vi "Main.vi"(11 "Module Admin":refnum<class "Delacor_lib_QMH_Module Admin.lvclass">) -> ()   [LabVIEW 2020, in "UI.lvlib"]
doc: "This template is based off of the Queued Message Handler design pattern and the Queued Message Handler project template that ships with LabVIEW.\n\nThe main difference is that the queue is private to this module and communication between modules is performed via Broadcast and Request events.\n\nRequest events are wrapped in public API methods and are handled in the Event Handling Loop (EHL) of this VI. Any module can register for Broadcast events sent by this module. The EHL generates messages based on user interface actions.\n\nThe Message Handling Loop (MHL) processes messages generated by the EHL, or by other messages. The messages are string values, so new messages can be added easily to the Message Cases case structure in the MHL. Each message cluster can also provide an optional value for Message Data, which is a variant that can be converted to whatever message-specific data is required.\n_____\nBased on DQMH Dev Tools: Project Template 7.1.1.1528."
uses:
  UI.lvlib
  <vilib>/Delacor/Delacor QMH/Libraries/Module Admin_class/Delacor_lib_QMH_Module Admin.lvclass
  <vilib>/Delacor/Delacor QMH/Libraries/Message Queue_class/Delacor_lib_QMH_Message Queue.lvclass/Delacor_lib_QMH_Message Queue.ctl
  <vilib>/Delacor/Delacor QMH/Libraries/Module Admin_class/Delacor_lib_QMH_Module Admin.lvclass/Delacor_lib_QMH_Module Admin.ctl
  <vilib>/Delacor/Delacor QMH/Libraries/Message Queue_class/Delacor_lib_QMH_Message Queue.lvclass
  Module Data--cluster.ctl
  <vilib>/Delacor/Delacor QMH/Libraries/Message Queue_class/Delacor_lib_QMH_Enqueue Message (Single).vi
  Stop Argument--cluster.ctl
  NI_DAQ/Libraries/NI DAQ/NI DAQ.lvlib
  NI_DAQ/Libraries/NI DAQ/Controls/AI config parameters--cluster.ctl
  <vilib>/Utility/sysdir.llb/System Directory Type.ctl
  <vilib>/Delacor/Delacor QMH/Libraries/Message Queue_class/Delacor_lib_QMH_Enqueue Message (Array).vi
panel:
  out "Remaining time":string caption="Tiempo restante"
  in  "Sample time":i32=1 caption="Muestreo (seg)"
  in  "Acq Time":dbl=1.0 caption="Tiempo (hrs)"
  in  "Log":bool
  in  "Stop Button":bool
  in  "Acquire":bool
  out "Temperatura":dbl format="%#_g °C"
  out "Voltage graph":dbl(graph)
  out "Status":string caption="Estado del sistema"
  out "Adquiriendo":bool
  out "DAQ":bool
  in  "Simulate MHL Error":bool
  in  "Simulate EHL Error":bool
  in  "Settings Button":bool
  in  "Exit Button":bool
  in  "Help Button":bool
  out "error out":errorcluster
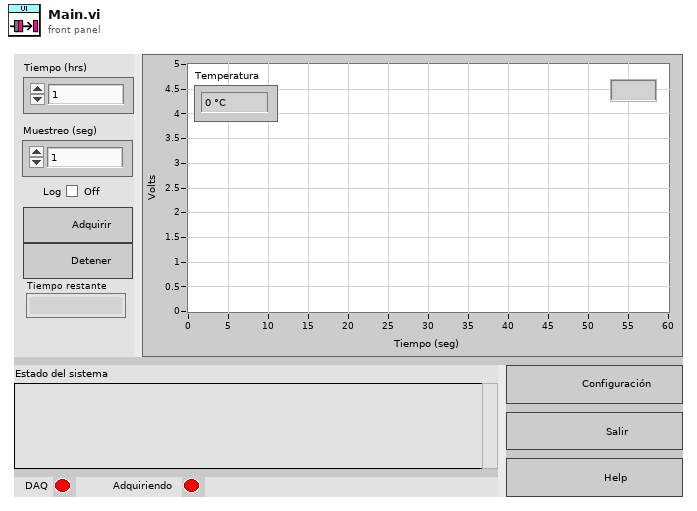
[diagram p1: front panel]
types:
  T1 = typedef "NI DAQ.lvlib/Broadcast Events--cluster.ctl" = cluster{"Module Did Init":refnum<user-event>, "Status Updated":refnum<user-event>, "Error Reported":refnum<user-event>, "Module Did Stop":refnum<user-event>, "Update Module Execution Status":refnum<user-event>, "Digital data acquired":refnum<user-event>, "Device connected":refnum<user-event>, "Connection failed":refnum<user-event>, "Analog data acquired":refnum<user-event>, "Counter data acquired":refnum<user-event>, "Temperature data acquired":refnum<user-event>}
  T2 = typedef "UI.lvlib/Request Events--cluster.ctl" = cluster{"Stop Module":refnum<user-event>, "Show Panel":refnum<user-event>, "Hide Panel":refnum<user-event>, "Get Module Execution Status":refnum<user-event>, "Show Diagram":refnum<user-event>}
  T3 = typedef "UI.lvlib/Module Data--cluster.ctl" = cluster{"Status":string, "DAQ module ID":i32, "DAQ Device":tag, "Start time":timestamp, "Stop time":timestamp, "Log file ref":refnum<file>}
  T4 = enum32{"invalid lock state", "Not Locked", "Locked (No Password)", "Password-protected"}
  T5 = typedef "UI.lvlib/Stop Argument--cluster.ctl" = cluster{"Origin":string, "Exit via Stop Module Req?":bool, "Wait for Module to stop?":bool}
  T6 = enum32{"Invalid", "Standard", "Closed", "Hidden", "Minimized", "Maximized"}
  T7 = cluster{"max value":dbl, "min value":dbl, "type":i32, "CJC source":i32, "cjc channel":refnum<k21>, "CJC value":dbl}
  T8 = typedef "NI DAQ.lvlib/AI config parameters--cluster.ctl" = cluster{"Terminal configuration":i32, "min value":dbl, "max value":dbl}
  T9 = enum16{"open", "replace", "create", "open or create", "replace or create", "replace or create with confirmation"}
  T10 = typedef "System Directory Type.ctl" = i32
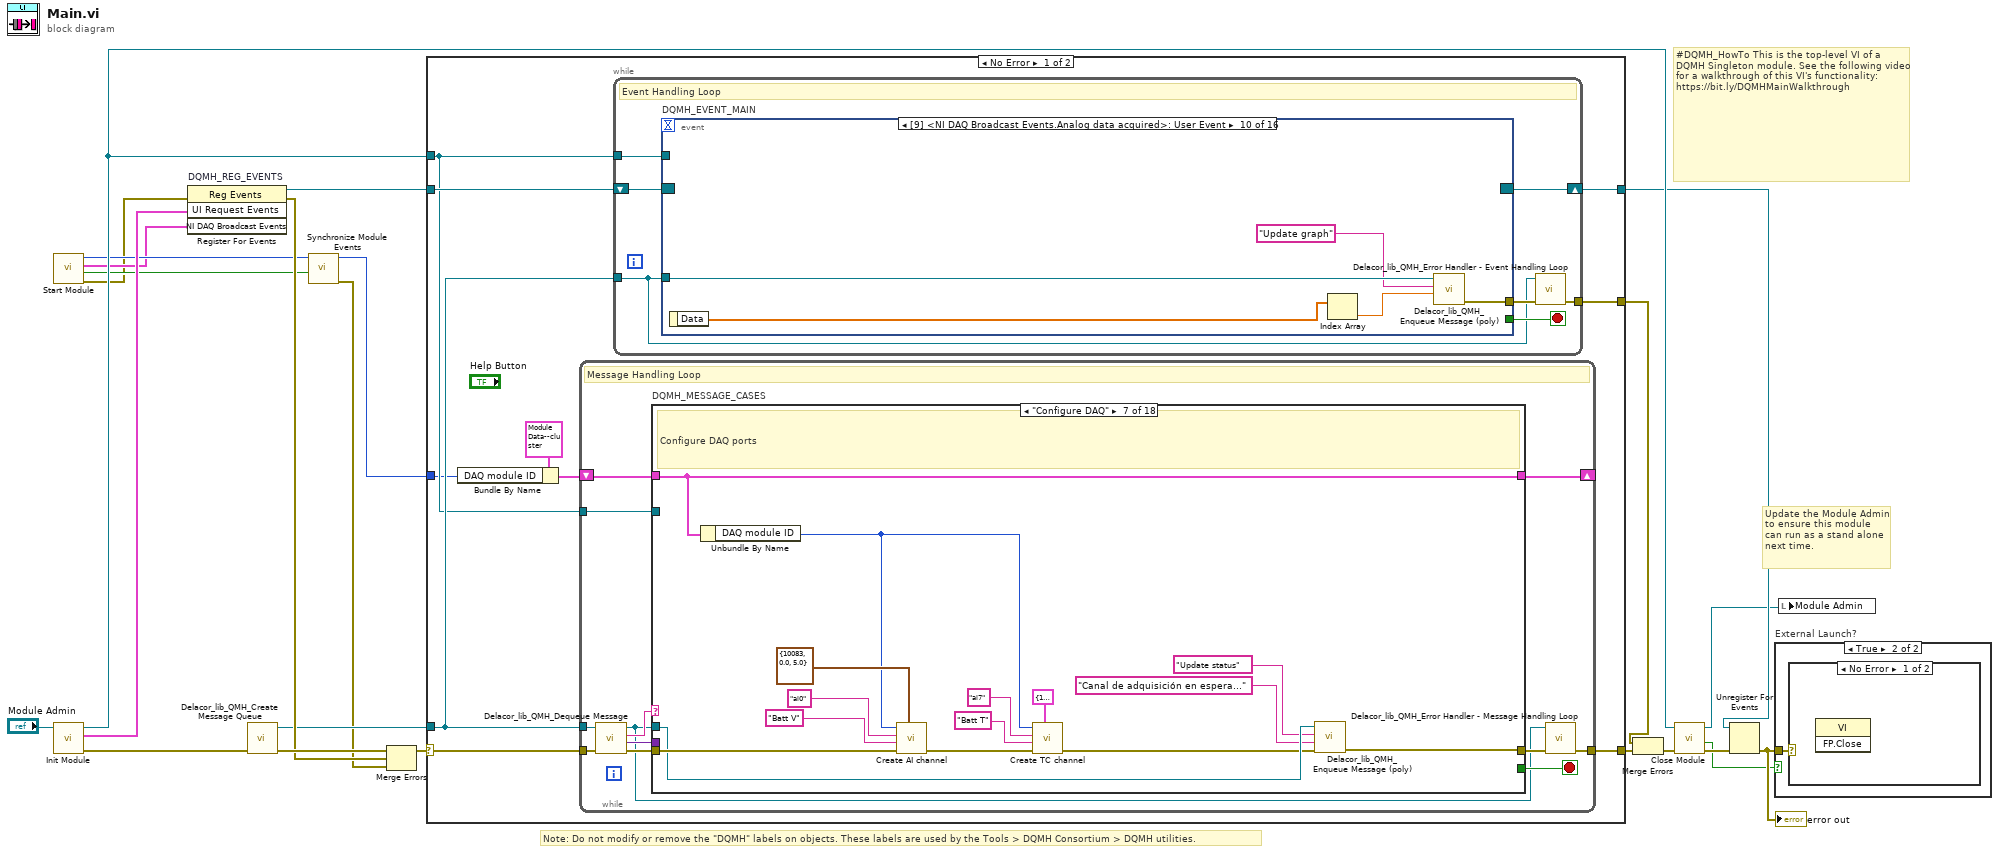
[diagram p0: block diagram]
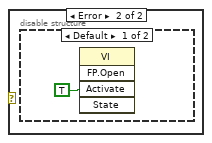
[diagram p3: hidden frame]
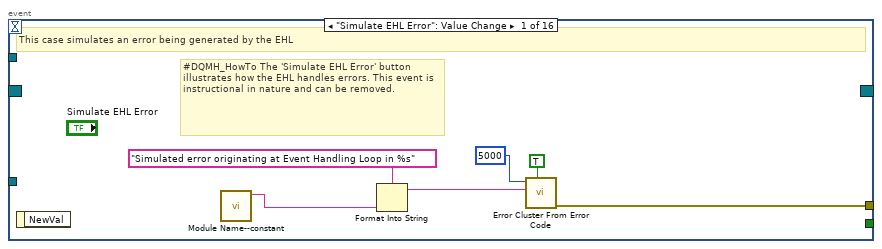
[diagram p5: hidden frame]
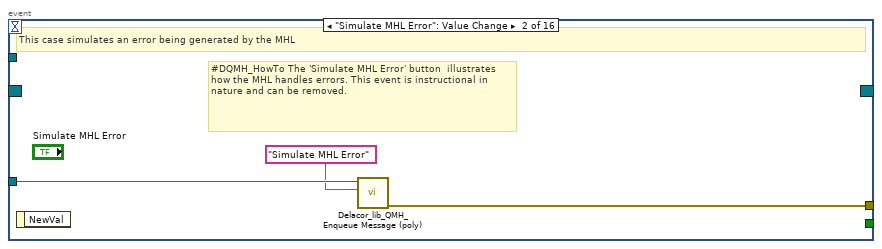
[diagram p6: hidden frame]
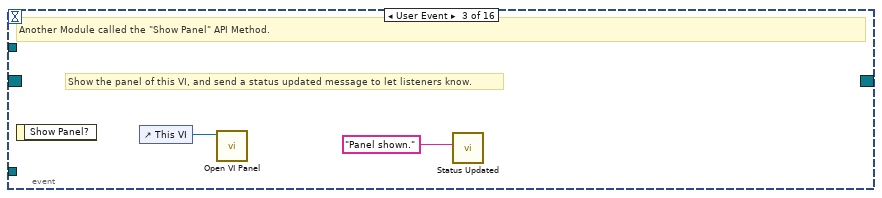
[diagram p7: hidden frame]
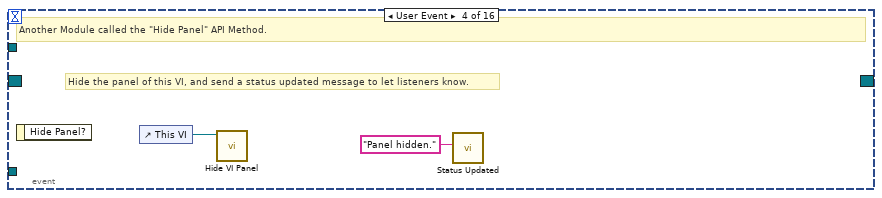
[diagram p8: hidden frame]
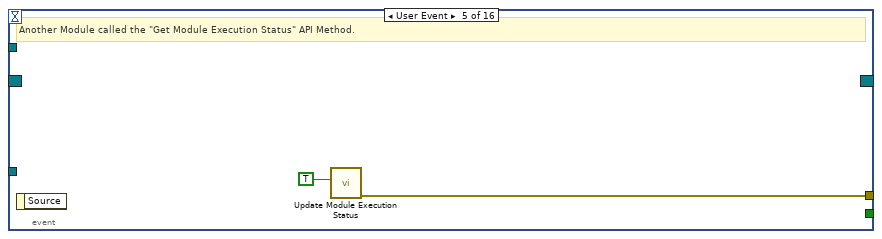
[diagram p9: hidden frame]
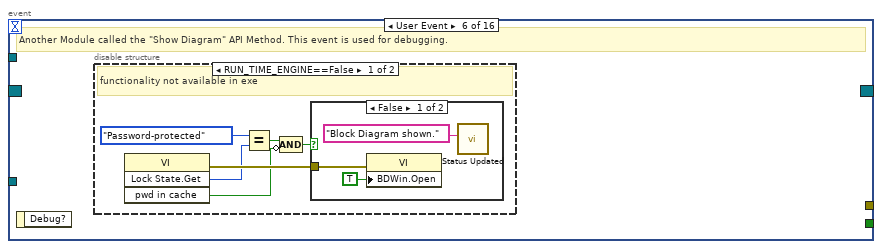
[diagram p10: hidden frame]
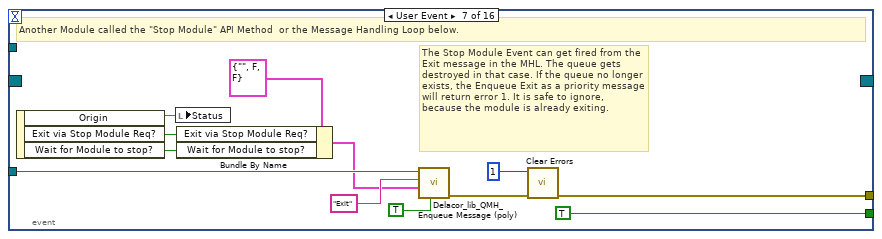
[diagram p13: hidden frame]
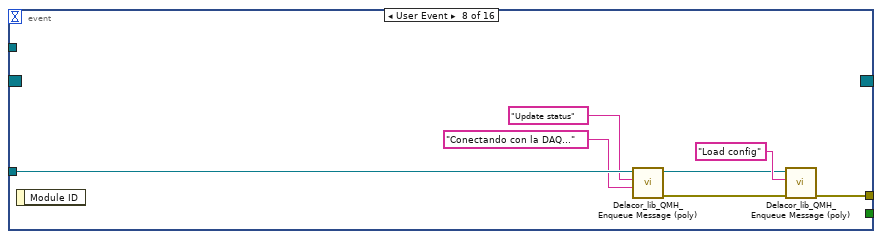
[diagram p14: hidden frame]
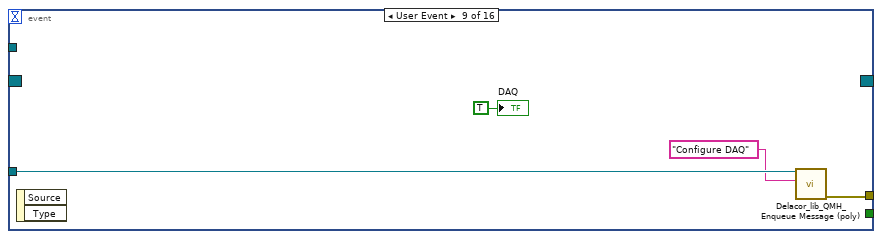
[diagram p15: hidden frame]
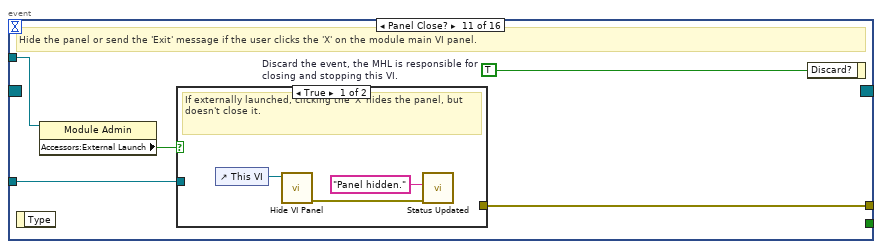
[diagram p16: hidden frame]
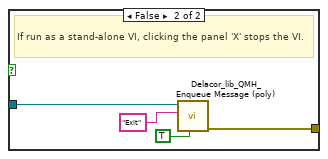
[diagram p17: hidden frame]
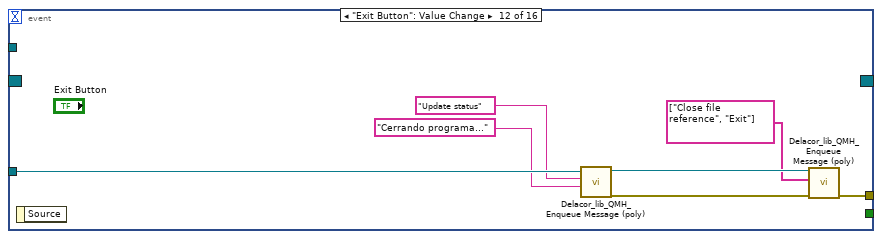
[diagram p18: hidden frame]
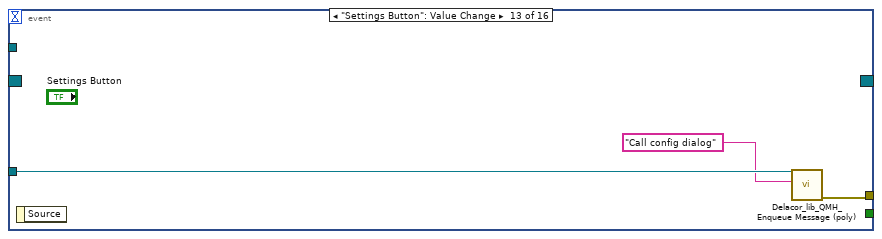
[diagram p19: hidden frame]
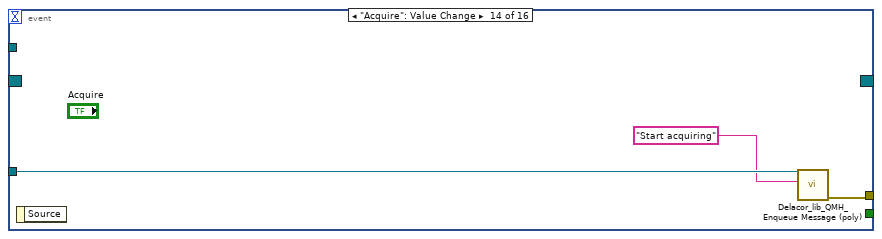
[diagram p20: hidden frame]
diagram:
  # "#DQMH_HowTo This is the top-level VI of a DQMH Singleton module. See the following video for a walkthrough of this VI's functionality: https://bit.ly/DQMHMainWalkthrough"
  # "Note: Do not modify or remove the \"DQMH\" labels on objects. These labels are used by the Tools > DQMH Consortium > DQMH utilities."
  # "Update the Module Admin to ensure this module can run as a stand alone next time."
  n1 = call "Start Module.vi"() -> ("error out"=w2:errorcluster, "Wait for Event Sync?"=w5:bool, "NI DAQ Broadcast Events"=w4:T1, "Module ID"=w6:i32)  [unwired: 8 in]
  n2 = call "Init Module.vi"("Singleton Module Admin in"="Module Admin") -> ("error out"=w22:errorcluster, "UI Request Events"=w11:T2, "Singleton Module Admin out"=w14:refnum<class "Delacor_lib_QMH_Module Admin.lvclass">)  [unwired: 8 in]
  n3 = register-events "DQMH_REG_EVENTS"(error in=w2, w11, w4) -> (reference out=w12:refnum<event-registration>, error out=w15:errorcluster)  [unwired: 1 in]
  n4 = call <vilib>:"Delacor_lib_QMH_Create Message Queue.vi"("error in"=w22) -> ("error out"=w17:errorcluster, "Message Queue"=w10:refnum<class "Delacor_lib_QMH_Message Queue.lvclass">)  [unwired: 9 in]
  n5 = call "Synchronize Module Events.vi"("Wait for Event Sync?"=w5, "Module ID in"=w6) -> ("error out"=w3:errorcluster, "Module ID out"=w1:i32)  [unwired: 8 in]
  n6 = Merge Errors(w17, w15, w3) -> (w16:errorcluster)
  n7 = case shown="No Error" w16 {
    selector: w16 -> [w31 w466]
    tunnel: [w33 w465] -> w23
    tunnel: [w30 w464] -> w13
    tunnel: w12 -> [w29 w464]
    tunnel: w10 -> [w28 w459]
    tunnel: [w32 _] -> w20
    tunnel: w14 -> [w27 w460]
    tunnel: w1 -> [w24 w458]
    frame No Error {
      n8 = Bundle By Name(cluster=T3 {"Status"="", "DAQ module ID"=0, "DAQ Device"="", "Start time"=timestamp(0 s since 1904-01-01), "Stop time"=timestamp(0 s since 1904-01-01), "Log file ref"=refnum} ("Data Cluster"), "DAQ module ID"=w24) -> (w26:T3)
      n9 = while {
        tunnel: w28 -> [w127]
        shift-right: [w135] -> _
        shift-left: w26 -> [w136]
        tunnel: w31 -> [w138]
        tunnel: [w130] -> w33
        tunnel: w27 -> [w131]
        stop <- w134 stop-if-true
        # "Message Handling Loop"
        n10 = call-dynamic "Delacor_lib_QMH_Dequeue Message.vi"("error in"=w138, "Message Queue in"=w127) -> ("error out"=w137:errorcluster, "Message Data"=w132:variant, "Message"=w133:string, "Message Queue out"=w128:refnum<class "Delacor_lib_QMH_Message Queue.lvclass">)  [unwired: 6 in]
        n11 = case "DQMH_MESSAGE_CASES" shown="\"Configure DAQ\"" w133 {
          selector: w133 -> [_ _ _ _ _ _ _ _ _ _ _ _ _ _ _ _ _ w453]
          tunnel: w128 -> [_ _ _ w176 w203 w221 w244 w264 w279 w296 w351 w380 _ _ _ w417 w441 _]
          tunnel: w137 -> [w162 w166 w169 w182 w204 w218 w250 w255 w274 w302 w355 w384 w396 w398 w413 w424 w447 w456]
          tunnel: [w161 w166 w168 w180 w198 w224 w245 w265 w280 w299 w352 w381 w389 w397 w412 w420 w442 w457] -> w129
          tunnel: w136 -> [w152 w165 w167 w181 w205 w220 w249 w267 w281 w286 w343 w383 w388 w399 w410 w419 w433 w454]
          tunnel: [w152 w165 w167 w170 w205 w219 w249 w266 w281 w286 w342 w383 w387 w399 w410 w419 w433 w454] -> w135
          tunnel: [_ _ _ _ _ _ _ _ _ _ _ _ _ _ _ _ w440 _] -> w134
          tunnel: w132 -> [_ _ _ _ _ _ _ _ _ w301 _ _ w394 _ _ w418 w439 _]
          tunnel: w131 -> [w153 _ _ _ _ _ _ _ _ _ _ _ _ _ _ w416 w434 _]
          frame "Initialize" {
            w140 = FALSE ("DAQ")
            # "Initialize - Any operation that needs to be done before the module can receive messages. Synchronize Caller Events.vi will inform Start Module.vi that the module has launched and is ready to receive messages. Module Did Init.vi will broadcast that the module initialized."
            n12 = call "Synchronize Caller Events.vi"("error in"=w162, "Singleton Module Admin in"=w153) -> ("error out"=w145:errorcluster, "Singleton Module Admin out"=w149:refnum<class "Delacor_lib_QMH_Module Admin.lvclass">)  [unwired: 8 in]
            n13 = property on="Property Node" class="Module Admin"(reference=w149) -> ("Accessors:External Launch"=w157:bool)  [unwired: 1 in, 2 out]
            n14 = property on="Voltage graph" class="WFChart (strict)"(error in=w145, "History Data"=dbl[] [], "XScale.RngStart"=0.0 ("X Scale.Range:Start"), "XScale.Maximum"=60.0 ("X Scale.Range:Maximum"), "XScale.Increment"=1.0 ("X Scale.Range:Increment")) -> (error out=w139:errorcluster)  [unwired: 1 in, 1 out]
            n15 = Select(t=T6."Hidden" ("State"), s=w157, f=T6."Standard" ("State")) -> (s? t:f=w154:T6)
            n16 = call "Module Name--constant.vi"() -> ("Module Name"=w160:string)  [unwired: 11 in]
            n17 = property on="Property Node" class="VI"("Front Panel.Title"=w160) -> (reference out=w159:refnum<vi>, error out=w164:errorcluster)  [unwired: 2 in]
            n18 = invoke on="Invoke Node" class="VI" method="FP.Open"(reference=w159, error in=w164, "State"=w154) -> (reference out=w158:refnum<vi>, error out=w163:errorcluster)  [unwired: 2 in, 3 out]
            n19 = property on="Adquiriendo" class="Bool (strict)"(error in=w139, "Value"=w140) -> ()  [unwired: 1 in, 2 out]
            n20 = property on="DAQ" class="Bool (strict)"(error in=w139, "Value"=w140) -> (error out=w148:errorcluster)  [unwired: 1 in, 1 out]
            n21 = control-ref of="This VI"() -> (w146:refnum<vi>)
            n22 = invoke on="Invoke Node" class="VI" method="FP.Center"(reference=w158, error in=w163) -> ()  [unwired: 1 in, 3 out]
            n23 = invoke class="VI" method="Default Vals.Reinit All"(reference=w146, error in=w148) -> (error out=w147:errorcluster)  [unwired: 1 in, 2 out]
            n24 = call "Module Name--constant.vi"() -> ("Module Name"=w150:string)  [unwired: 11 in]
            n25 = call "Module Did Init.vi"("error in"=w147, "Initialized?"=TRUE, "Origin"=w150) -> ("error out"=w161:errorcluster)  [unwired: 8 in]
          }
          frame "---Module Specific---" {
            # "Separator -- The following cases handle messages specific to this Module."
          }
          frame "---Copy This Frame---" {
            # "Duplicate this frame when creating new messages.  Change this comment in the duplicated frame to describe this message."
            n26 = Merge Errors(w169) -> (w168:errorcluster)
          }
          frame "Load config" {
            # "Try to load data from config.ini. If file is non existent, call configuration dialog, otherwise configure DAQ and enter idle status."
            n27 = call "Load config.vi"("error in (no error)"=w182, "Data Cluster in"=w181) -> ("error out"=w172:errorcluster, "Call config dialog?"=w179:bool, "Data Cluster out"=w170:T3)  [unwired: 7 in]
            n28 = case shown="True" w179 {
              tunnel: ["Validate DAQ" "Call config dialog"] -> w178
              tunnel: ["Configuración cargada. Validando..." "DAQ no conectada. Lanzando diálogo de configuración."] -> w173
              tunnel: w172 -> [w187 w192]
              tunnel: [w186 w191] -> w171
              tunnel: w170 -> [w185 _]
              frame False {
                # "Connection successful. Validate DAQ."
                n29 = Unbundle By Name(w185) -> ("DAQ module ID"=w184:i32, "DAQ Device"=w183:tag)
                n30 = call "Set device name.vi"("error in"=w187, "Device name"=w183, "Module ID"=w184) -> ("error out"=w186:errorcluster)  [unwired: 8 in]
              }
              frame True {
                w190 = -200220  # Invalid DAQ name reference
                # "Connection failed. Send config dialog"
                n31 = call <vilib>:"Clear Errors.vi"("error in (no error)"=w192, "specific error code to clear (0: all)"=w190) -> ("error out"=w191:errorcluster)  [unwired: 4 in, 1 out]
              }
            }
            n32 = call-poly <vilib>:"Delacor_lib_QMH_Enqueue Message (poly).vi"("error in"=w171, "Message Data"=w173, "Message"="Update status", "Message Queue in"=w176) -> ("error out"=w177:errorcluster, "Message Queue out"=w175:refnum<class "Delacor_lib_QMH_Message Queue.lvclass">)  [unwired: 6 in]
            n33 = call-poly <vilib>:"Delacor_lib_QMH_Enqueue Message (poly).vi"("error in"=w177, "Message"=w178, "Message Queue in"=w175) -> ("error out"=w180:errorcluster)  [unwired: 7 in, 1 out]
          }
          frame "Validate DAQ" {
            # "Identify DAQ Model and validate connection."
            n34 = Unbundle By Name(w205) -> ("DAQ module ID"=w195:i32)
            n35 = call "Get device model.vi"("error in"=w204, "Module ID"=w195) -> ("error out"=w197:errorcluster, "Device model"=w200:string)  [unwired: 7 in, 1 out]
            n36 = Empty String/Path?(string/path=w200) -> (empty?=w199:bool)
            n37 = case shown="False" w199 {
              tunnel: [w210 "La tarjeta DAQ conectada no es válida."] -> w201
              tunnel: w200 -> [w209 _]
              tunnel: w197 -> [w208 w213]
              tunnel: [w207 w213] -> w196
              tunnel: w195 -> [w206 _]
              frame False {
                # "DAQ Model not empty. Validate connection."
                n38 = Format Into String(format string="DAQ %s encontrada.", w209) -> (resulting string=w210:string)  [unwired: 2 in, 1 out]
                n39 = call "Validate connection.vi"("error in"=w208, "Module ID"=w206) -> ("error out"=w207:errorcluster)  [unwired: 7 in, 2 out]
              }
              frame True {
                # "DAQ Model string empty."
              }
            }
            n40 = call-poly <vilib>:"Delacor_lib_QMH_Enqueue Message (poly).vi"("error in"=w196, "Message Data"=w201, "Message"="Update status", "Message Queue in"=w203) -> ("error out"=w198:errorcluster)  [unwired: 6 in, 1 out]
          }
          frame "Call config dialog" {
            n41 = property on="DAQ" class="Bool (strict)"(error in=w218, "Value"=FALSE ("DAQ")) -> (error out=w216:errorcluster)  [unwired: 1 in, 1 out]
            n42 = Unbundle By Name(w220) -> ("DAQ module ID"=w214:i32)
            n43 = call "Stop continuous acquisition.vi"("error in"=w216, "Module ID"=w214) -> ("error out"=w215:errorcluster)  [unwired: 9 in]
            n44 = call "Config dialog.vi"("error in (no error)"=w215, "DAQ module ID"=w214) -> ("error out"=w225:errorcluster, "Cancelled?"=w223:bool, "DAQmx Device Name out"=w222:tag)  [unwired: 7 in]
            n45 = case shown="False" w223 {
              tunnel: w225 -> [w227 w235]
              tunnel: [w233 w235] -> w224
              tunnel: w222 -> [w228 _]
              tunnel: w221 -> [w232 _]
              tunnel: w220 -> [w230 w234]
              tunnel: [w229 w234] -> w219
              frame False {
                # "Save config and try to connect."
                n46 = call "Save config.vi"("error in (no error)"=w227, "DAQ Device Name"=w228) -> ("error out"=w226:errorcluster)  [unwired: 9 in]
                n47 = Bundle By Name(cluster=w230, "DAQ Device"=w228) -> (w229:T3)
                n48 = call-poly <vilib>:"Delacor_lib_QMH_Enqueue Message (poly).vi"("error in"=w226, "Message"="Load config", "Message Queue in"=w232) -> ("error out"=w233:errorcluster)  [unwired: 7 in, 1 out]
              }
              frame True {
                # "Dialog was cancelled. Do nothing."
              }
            }
          }
          frame "Configure DAQ" {
            # "Configure DAQ ports"
            n49 = Unbundle By Name(w249) -> ("DAQ module ID"=w239:i32)
            n50 = call "Create AI channel.vi"("Config params"=T8 {"Terminal configuration"=10083, "min value"=0.0, "max value"=5.0}, "error in"=w250, "Channel name"="Batt V", "Physical channel"="ai0", "Module ID"=w239) -> ("error out"=w241:errorcluster)  [unwired: 6 in]
            n51 = call "Create TC channel.vi"("TC Config"=T7 {"max value"=100.0, "min value"=0.0, "type"=10073, "CJC source"=10116, "cjc channel"="", "CJC value"=23.0}, "error in"=w241, "Channel name"="Batt T", "Physical channel"="ai7", "Module ID"=w239) -> ("error out"=w240:errorcluster)  [unwired: 6 in]
            n52 = call-poly <vilib>:"Delacor_lib_QMH_Enqueue Message (poly).vi"("error in"=w240, "Message Data"="Canal de adquisición en espera..." ("Message"), "Message"="Update status", "Message Queue in"=w244) -> ("error out"=w245:errorcluster)  [unwired: 6 in, 1 out]
          }
          frame "Start acquiring" {
            w270 = 1000  # To ms
            # "Begin continuous acquisition of analog input channel."
            n53 = Unbundle By Name(w267) -> ("DAQ module ID"=w252:i32)
            n54 = Multiply(x="Sample time", y=w270) -> (x*y=w251:i32)
            n55 = call "Start continuous AI.vi"("error in"=w255, "Acq type"=enum16{"Single", "Multiple"}."Single" ("Samples"), "Timeout"=w251, "Module ID"=w252) -> ("error out"=w253:errorcluster)  [unwired: 7 in]
            n56 = local read "Acq Time"() -> (w260:dbl)
            n57 = Get Date/Time In Seconds() -> (seconds since 1Jan1904=w258:timestamp)
            n58 = property on="Voltage graph" class="WFChart (strict)"(error in=w253, "History Data"=dbl[] []) -> (error out=w269:errorcluster)  [unwired: 1 in, 1 out]
            n59 = Multiply(x=w260, y=3600.0) -> (x*y=w257:dbl)
            n60 = Add(x=w258, y=w257) -> (x+y=w256:timestamp)
            n61 = Bundle By Name(cluster=w267, "Start time"=w258, "Stop time"=w256) -> (w266:T3)
            n62 = call-poly <vilib>:"Delacor_lib_QMH_Enqueue Message (poly).vi"("error in"=w269, "Message Data"="Adquisición en progreso..." ("Message"), "Message"="Update status", "Message Queue in"=w264) -> ("error out"=w265:errorcluster)  [unwired: 6 in, 1 out]
            "Adquiriendo" <- TRUE ("Adquiriendo")
          }
          frame "Stop acquisition" {
            n63 = Unbundle By Name(w281) -> ("DAQ module ID"=w272:i32)
            n64 = call "Stop continuous AI.vi"("error in"=w274, "Module ID"=w272) -> ("error out"=w273:errorcluster)  [unwired: 9 in]
            n65 = property on="Adquiriendo" class="Bool (strict)"(error in=w273, "Value"=FALSE ("Adquiriendo")) -> (error out=w276:errorcluster)  [unwired: 1 in, 1 out]
            n66 = call-poly <vilib>:"Delacor_lib_QMH_Enqueue Message (poly).vi"("error in"=w276, "Message Data"="Adquisitión detenida" ("Message"), "Message"="Update status", "Message Queue in"=w279) -> ("error out"=w280:errorcluster)  [unwired: 6 in, 1 out]
          }
          frame "Update graph" {
            w293 = 3600.0  # h to sec
            # "Updates graph contents and checks wether Log to file is active. If Log is set to True, write a new row to Log file."
            n67 = Variant To Data(error in=w302, type=0.0, Variant=w301) -> (data=w294:dbl, error out=w288:errorcluster)
            "Voltage graph" <- w294
            n68 = Unbundle By Name(w286) -> ("Stop time"=w289:timestamp, "Start time"=w290:timestamp)
            n69 = Unbundle By Name(w286) -> ("DAQ module ID"=w285:i32)
            n70 = Get Date/Time In Seconds() -> (seconds since 1Jan1904=w295:timestamp)
            n71 = Subtract(x=w295, y=w290) -> (x-y=w298:dbl)
            n72 = call "Read TC.vi"("error in"=w288, "N samples"=10, "Reading Type"=enum16{"Single", "Average"}."Average", "Module ID"=w285) -> ("error out"=w287:errorcluster, "Temperature"=w282:dbl)  [unwired: 5 in, 1 out]
            "Temperatura" <- w282
            n73 = Multiply(x="Acq Time", y=w293) -> (x*y=w291:dbl)
            n74 = Less Or Equal?(x=w298, y=w291) -> (x <= y?=w297:bool)
            n75 = case shown="True" w297 {
              tunnel: w287 -> [w304 w327]
              tunnel: [w308 w325] -> w299
              tunnel: w286 -> [w318 w324]
              tunnel: w296 -> [w314 _]
              tunnel: w295 -> [w311 w322]
              tunnel: w294 -> [_ w323]
              tunnel: w289 -> [_ w321]
              tunnel: w282 -> [_ w319]
              frame False {
                # "Total acquisition time reached. Stop acquisition"
                n76 = Unbundle By Name(w318) -> ("DAQ module ID"=w317:i32)
                n77 = property on="Adquiriendo" class="Bool (strict)"(error in=w304, "Value"=FALSE ("Adquiriendo")) -> (error out=w303:errorcluster)  [unwired: 1 in, 1 out]
                n78 = Format Date/Time String(seconds (now)=w311) -> (date/time string=w310:string)  [unwired: 2 in]
                n79 = call "Stop continuous acquisition.vi"("error in"=w303, "Module ID"=w317) -> ("error out"=w316:errorcluster)  [unwired: 9 in]
                n80 = Format Into String(format string="Adquisición completada en %s.", w310) -> (resulting string=w309:string)  [unwired: 2 in, 1 out]
                n81 = One Button Dialog(message=w309) -> ()  [unwired: 1 in, 1 out]
                n82 = call-poly <vilib>:"Delacor_lib_QMH_Enqueue Message (poly).vi"("error in"=w316, "Message Data"=w309, "Message"="Update status", "Message Queue in"=w314) -> ("error out"=w315:errorcluster, "Message Queue out"=w307:refnum<class "Delacor_lib_QMH_Message Queue.lvclass">)  [unwired: 6 in]
                n83 = call-poly <vilib>:"Delacor_lib_QMH_Enqueue Message (poly).vi"("error in"=w315, "Message"="Close file reference", "Message Queue in"=w307) -> ("error out"=w308:errorcluster)  [unwired: 7 in, 1 out]
              }
              frame True {
                # "Total acquisition time not reached yet. Keep acquiring."
                n84 = call "Get remaining time.vi"("Stop time"=w321, "Curent time"=w322) -> ("Remaining time"=→"Remaining time":string)  [unwired: 9 in]
                n85 = case shown="True" "Log" {
                  tunnel: w327 -> [w328 w341]
                  tunnel: [w328 w336] -> w325
                  tunnel: w324 -> [_ w340]
                  tunnel: w323 -> [_ w331]
                  tunnel: w322 -> [_ w339]
                  tunnel: w319 -> [_ w329]
                  frame False {
                    # "Not logging. Do nothing."
                  }
                  frame True {
                    # "Log to file"
                    n86 = Unbundle By Name(w340) -> ("Log file ref"=w334:refnum<file>)
                    n87 = Get Date/Time String(date format (0)=enum16{"short", "long", "abbreviated"}."short", seconds (now)=w339, want seconds? (F)=TRUE) -> (date string=w333:string, time string=w332:string)
                    n88 = Format Into String(format string="%s %s,%0.6f,%0.2f\n", w333, w332, w331, w329) -> (resulting string=w335:string)  [unwired: 2 in, 1 out]
                    n89 = Write to Text File(file (use dialog)=w334, text=w335, error in=w341) -> (error out=w336:errorcluster)  [unwired: 1 in, 2 out]
                  }
                }
              }
            }
          }
          frame "Open file reference" {
            w347 = T10 2 items=["User Home"=0, "User Desktop"=1, "User Documents"=2, "User Application Data"=3, "User Preferences"=4, "User Temporary"=5, "Public Documents"=6, "Public Application Data"=7, "Public Preferences"=8, "Public Cache"=13, "System Core Libraries"=9, "System Installed Libraries"=10, "Application Files"=11, "Boot Volume Root"=12] ("system directory type")
            n90 = call <vilib>:"Get System Directory.vi"("system directory type"=w347) -> ("system directory"=w346:path)  [unwired: 10 in]
            n91 = call "File Dialog"("start path"=w346, "error in"=w355, "pattern (all files)"="*.csv") -> ("selected path"=w345:path, "cancelled"=w354:bool, "error out"=w344:errorcluster)  [unwired: 9 in, 1 out]
            n92 = case shown="False" w354 {
              tunnel: [w359 w374] -> w353
              tunnel: ["Registro de datos iniciado." ("Message") "Registro de datos cancelado." ("Message")] -> w349
              tunnel: w345 -> [w366 _]
              tunnel: w344 -> [w367 w369]
              tunnel: w343 -> [w361 w371]
              tunnel: [w360 w371] -> w342
              frame False {
                # "Dialog not cancelled. Open file reference."
                n93 = Open/Create/Replace File(file path (use dialog)=w366, error in=w367, operation (0:open)=T9."replace or create", access (0:read/write)=enum16{"read/write", "read-only", "write-only"}."write-only") -> (refnum out=w358:refnum<file>, error out=w365:errorcluster)  [unwired: 2 in, 1 out]
                n94 = Write to Text File(file (use dialog)=w358, text="Timestamp,Voltaje, Temperatura\n", error in=w365) -> (refnum out=w356:refnum<file>, error out=w359:errorcluster)  [unwired: 1 in, 1 out]
                n95 = Bundle By Name(cluster=w361, "Log file ref"=w356) -> (w360:T3)
              }
              frame True {
                w370 = 43  # Dialog cancelled
                # "Dialog was cancelled. Set Log flag to False."
                n96 = call <vilib>:"Clear Errors.vi"("error in (no error)"=w369, "specific error code to clear (0: all)"=w370) -> ("error out"=w368:errorcluster)  [unwired: 4 in, 1 out]
                n97 = property on="Log" class="Bool (strict)"(error in=w368, "Value"=FALSE ("Log")) -> (error out=w374:errorcluster)  [unwired: 1 in, 1 out]
              }
            }
            n98 = call-poly <vilib>:"Delacor_lib_QMH_Enqueue Message (poly).vi"("error in"=w353, "Message Data"=w349, "Message"="Update status", "Message Queue in"=w351) -> ("error out"=w352:errorcluster)  [unwired: 6 in, 1 out]
          }
          frame "Close file reference" {
            w377 = 1  # Log file not initiated, ignore.
            n99 = Unbundle By Name(w383) -> ("Log file ref"=w382:refnum<file>)
            n100 = Close File(refnum=w382, error in=w384) -> (error out=w376:errorcluster)  [unwired: 1 out]
            n101 = call <vilib>:"Clear Errors.vi"("error in (no error)"=w376, "specific error code to clear (0: all)"=w377) -> ("error out"=w375:errorcluster)  [unwired: 4 in, 1 out]
            n102 = call-poly <vilib>:"Delacor_lib_QMH_Enqueue Message (poly).vi"("error in"=w375, "Message Data"="Registro de datos detenido." ("Message"), "Message"="Update status", "Message Queue in"=w380) -> ("error out"=w381:errorcluster)  [unwired: 6 in, 1 out]
          }
          frame "Update status" {
            # "Updates the status indicator in the FP and creates a historic buffer of messages sent to indicator."
            n103 = Variant To Data(error in=w396, type="", Variant=w394) -> (data=w391:string, error out=w390:errorcluster)
            n104 = Unbundle By Name(w388) -> ("Status"=w393:string)
            n105 = Format Into String(format string="\n%s", initial string=w393, w391) -> (resulting string=w386:string)  [unwired: 1 in, 1 out]
            n106 = property on="Status" class="Str"(error in=w390, "Value"=w386, "Text.Scroll Position"=u32 2000) -> (error out=w389:errorcluster)  [unwired: 1 in, 1 out]
            n107 = Bundle By Name(cluster=w388, "Status"=w386) -> (w387:T3)
          }
          frame "---Exit and Error Handling---" {
            # "Separator - The following cases handle errors and exit messages."
            n108 = case shown="Error 1" w398 {
              selector: w398 -> [w400 w403 w404]
              tunnel: [w400 w402 w404] -> w397
              frame No Error {
              }
              frame Error {
                w401 = 1  # Log file not initiated, ignore.
                n109 = call <vilib>:"Clear Errors.vi"("error in (no error)"=w403, "specific error code to clear (0: all)"=w401) -> ("error out"=w402:errorcluster)  [unwired: 4 in, 1 out]
              }
              frame Default {
              }
            }
          }
          frame "Simulate MHL Error" {
            # "#DQMH_HowTo The 'Simulate MHL Error' button  illustrates how the MHL handles errors. This event is instructional in nature and can be removed."
            # "Simulate an error occurring at the MHL"
            n110 = call "Module Name--constant.vi"() -> ("Module Name"=w406:string)  [unwired: 11 in]
            n111 = Format Into String(format string="Simulated error originating at Message Handling Loop in %s", w406) -> (resulting string=w407:string)  [unwired: 2 in, 1 out]
            n112 = call <vilib>:"Error Cluster From Error Code.vi"("show call chain? (False)"=TRUE, "error message (\"\")"=w407, "error code (0)"=5001) -> ("error out"=w411:errorcluster)  [unwired: 6 in]
            n113 = Merge Errors(w413, w411) -> (w412:errorcluster)
          }
          frame "Error" {
            # "#DQMH_CodeRecommended - If the module is running in standalone mode (External Launch = FALSE), this code will pop up an error dialog and call the 'Exit' message if an error occurs. Add more fine-grained error management here."
            # "Error - Check the error message data and respond accordingly. This message is sent by the \"Error Handler\" VIs at the end of each loop in this application."
            n114 = property on="Property Node" class="Module Admin"(reference=w416) -> ("Accessors:External Launch"=w415:bool)  [unwired: 1 in, 2 out]
            n115 = Variant To Data(error in=w424, type=errorcluster {"status"=FALSE, "code"=0, "source"=""} ("error constant"), Variant=w418) -> (data=w414:errorcluster, error out=w422:errorcluster)
            n116 = local write "error out"(w414) -> ()
            n117 = call "Error Reported.vi"("Error"=w414) -> ()  [unwired: 10 in, 1 out]
            n118 = case shown="False" w415 {
              tunnel: [w429 _] -> w421
              tunnel: w417 -> [w427 _]
              tunnel: w414 -> [w428 _]
              frame False {
                n119 = disable-structure shown="Default" {
                  disable-tunnel: w428 -> [w430 _]
                  frame condition #0 (active) {
                    # "If the module is running standalone, then pop up an error dialog and call the \"Exit\" message."
                    n120 = call <vilib>:"Simple Error Handler.vi"("error in (no error)"=w430) -> ()  [unwired: 4 in, 5 out]
                  }
                  frame condition #1 {
                    # "To prevent the Simple Error Handler VI from being loaded (e.g. when deploying to a Real-Time target), add the Conditional Disable Symbol \"DQMH_Disable_SEH\" to your project and set it to TRUE."
                  }
                }
                n121 = call-poly <vilib>:"Delacor_lib_QMH_Enqueue Message (poly).vi"("Priority Message? (F)"=TRUE, "Message"="Exit", "Message Queue in"=w427) -> ("error out"=w429:errorcluster)  [unwired: 7 in, 1 out]
              }
              frame True {
                # "If the module was launched externally, calling the Error Reported broadcast VI is the only action performed by the \"Error\" message. The module's caller can then process the error appropriately."
              }
            }
            n122 = Merge Errors(w422, w421) -> (w420:errorcluster)
          }
          frame "Exit" {
            w438 = 91  # 91: not all Exit messages will have an argument
            w440 = TRUE  # Stop the VI
            # "Release the message queue reference"
            # "Exit - Exit the application."
            n123 = Variant To Data(error in=w447, type=T5 {"Origin"="", "Exit via Stop Module Req?"=FALSE, "Wait for Module to stop?"=FALSE} ("Stop Argument"), Variant=w439) -> (data=w436:T5, error out=w444:errorcluster)
            n124 = Unbundle By Name(w433) -> ("DAQ module ID"=w431:i32)
            n125 = call <vilib>:"Clear Errors.vi"("error in (no error)"=w444, "specific error code to clear (0: all)"=w438) -> ("error out"=w446:errorcluster)  [unwired: 4 in, 1 out]
            n126 = call "Stop continuous AI.vi"("Module ID"=w431) -> ("error out"=w432:errorcluster)  [unwired: 10 in]
            n127 = control-ref of="This VI"() -> (w435:refnum<vi>)
            n128 = call-dynamic "Delacor_lib_QMH_Release Message Queue.vi"("error in"=w446, "Message Queue"=w441) -> ("error out"=w445:errorcluster)  [unwired: 9 in]
            n129 = call "Handle Exit.vi"("Stop Argument"=w436, "Admin in"=w434, "VI reference"=w435) -> ("error out"=w443:errorcluster)  [unwired: 7 in, 1 out]
            n130 = call "Stop Module.vi"("error in"=w432, "Module ID"=w431) -> ()  [unwired: 9 in, 1 out]
            n131 = Merge Errors(w445, w443) -> (w442:errorcluster)
            n132 = call "Error Reported.vi"("Error"=w442) -> ()  [unwired: 10 in, 1 out]
          }
          frame Default {
            # "'Default' case only runs if there is a message that isn't defined in any of the other cases.  Output a programming error."
            n133 = call "Module Name--constant.vi"() -> ("Module Name"=w452:string)  [unwired: 11 in]
            n134 = Format Into String(format string="The invalid message string \"%s\" was received in the Message Handling Loop for module \"%s\".", w453, w452) -> (resulting string=w448:string)  [unwired: 2 in, 1 out]
            n135 = call <vilib>:"Error Cluster From Error Code.vi"("show call chain? (False)"=TRUE, "error message (\"\")"=w448, "error code (0)"=1) -> ("error out"=w455:errorcluster)  [unwired: 6 in]
            n136 = Merge Errors(w456, w455) -> (w457:errorcluster)
          }
        }
        n137 = call-dynamic "Delacor_lib_QMH_Error Handler - Message Handling Loop.vi"("error in"=w129, "Message Queue in"=w128) -> ("dup error in"=w130:errorcluster)  [unwired: 8 in, 1 out]
      }
      n138 = while {
        tunnel: w28 -> [w34]
        shift-right: [w37] -> w30
        shift-left: w29 -> [w38]
        tunnel: [w39] -> w32
        tunnel: w27 -> [w35]
        stop <- w36 stop-if-true
        # "Event Handling Loop"
        n139 = event "DQMH_EVENT_MAIN" shown="[9] <NI DAQ Broadcast Events.Analog data acquired>: User Event" {
          selector: w38 -> [_ _ _ _ _ _ _ _ _ _ _ _ _ _ _ _]
          dyn-events: [_ _ _ _ _ _ _ _ _ _ _ _ _ _ _ _] -> w37
          timeout: _ -> [_ _ _ _ _ _ _ _ _ _ _ _ _ _ _ _]
          tunnel: [_ _ _ _ _ _ TRUE ("Discard?") _ _ _ _ _ _ _ _ _] -> w36
          tunnel: w34 -> [_ w48 _ _ _ _ w72 w80 w86 w91 w95 w110 w113 w116 w119 w122]
          tunnel: [w46 w49 _ _ w55 _ w75 w83 w87 w92 w97 w111 w114 w117 w120 w123] -> w40
          tunnel: w35 -> [_ _ _ _ _ _ _ _ _ _ w94 _ _ _ _ _]
          event "Simulate EHL Error": Value Change {
            # "#DQMH_HowTo The 'Simulate EHL Error' button  illustrates how the EHL handles errors. This event is instructional in nature and can be removed."
            # "This case simulates an error being generated by the EHL"
            n140 = event-data() -> ()  [unwired: 1 in, 1 out]
            n141 = call "Module Name--constant.vi"() -> ("Module Name"=w43:string)  [unwired: 11 in]
            n142 = Format Into String(format string="Simulated error originating at Event Handling Loop in %s", w43) -> (resulting string=w44:string)  [unwired: 2 in, 1 out]
            n143 = call <vilib>:"Error Cluster From Error Code.vi"("show call chain? (False)"=TRUE, "error message (\"\")"=w44, "error code (0)"=5000) -> ("error out"=w46:errorcluster)  [unwired: 6 in]
          }
          event "Simulate MHL Error": Value Change {
            # "#DQMH_HowTo The 'Simulate MHL Error' button  illustrates how the MHL handles errors. This event is instructional in nature and can be removed."
            # "This case simulates an error being generated by the MHL"
            n144 = event-data() -> ()  [unwired: 1 in, 1 out]
            n145 = call-poly <vilib>:"Delacor_lib_QMH_Enqueue Message (poly).vi"("Message"="Simulate MHL Error", "Message Queue in"=w48) -> ("error out"=w49:errorcluster)  [unwired: 8 in, 1 out]
          }
          event User Event {
            # "Show the panel of this VI, and send a status updated message to let listeners know."
            # "Another Module called the \"Show Panel\" API Method."
            n146 = event-data() -> ()  [unwired: 1 in, 1 out]
            n147 = control-ref of="This VI"() -> (w51:refnum<vi>)
            n148 = call "Open VI Panel.vi"("VI"=w51) -> ()  [unwired: 10 in, 1 out]
            n149 = call "Status Updated.vi"("Status"="Panel shown." ("format string")) -> ()  [unwired: 10 in, 1 out]
          }
          event User Event {
            # "Hide the panel of this VI, and send a status updated message to let listeners know."
            # "Another Module called the \"Hide Panel\" API Method."
            n150 = event-data() -> ()  [unwired: 1 in, 1 out]
            n151 = control-ref of="This VI"() -> (w53:refnum<vi>)
            n152 = call "Hide VI Panel.vi"("VI"=w53) -> ()  [unwired: 10 in, 1 out]
            n153 = call "Status Updated.vi"("Status"="Panel hidden." ("format string")) -> ()  [unwired: 10 in, 1 out]
          }
          event User Event {
            # "Another Module called the \"Get Module Execution Status\" API Method."
            n154 = event-data() -> ()  [unwired: 1 in, 1 out]
            n155 = call "Update Module Execution Status.vi"("Running?"=TRUE) -> ("error out"=w55:errorcluster)  [unwired: 10 in]
          }
          event User Event {
            # "Another Module called the \"Show Diagram\" API Method. This event is used for debugging."
            n156 = event-data() -> ()  [unwired: 1 in, 1 out]
            n157 = disable-structure shown="RUN_TIME_ENGINE==False" {
              frame condition #0 (active) {
                # "functionality not available in exe"
                n158 = invoke on="Invoke Node" class="VI" method="Lock State.Get"() -> (error out=w61:errorcluster, "Get Lock State"=w60:T4, "pwd in cache"=w57:bool)  [unwired: 4 in, 1 out]
                n159 = Equal?(x=T4."Password-protected", y=w60) -> (x = y?=w58:bool)
                n160 = Compound Arithmetic op=AND(w58, invert w57) -> (w56:bool)
                n161 = case shown="False" w56 {
                  tunnel: w61 -> [w64 _]
                  frame False {
                    n162 = property on="Property Node" class="VI"(error in=w64, "BDWin.Open"=TRUE ("Block Diagram Window:Open")) -> ()  [unwired: 1 in, 2 out]
                    n163 = call "Status Updated.vi"("Status"="Block Diagram shown." ("format string")) -> ()  [unwired: 10 in, 1 out]
                  }
                  frame True {
                    # "Password-protected VI, and the password is not in the cache. Do not show the diagram."
                  }
                }
              }
              frame condition #1 {
              }
            }
          }
          event User Event {
            # "The Stop Module Event can get fired from the Exit message in the MHL. The queue gets destroyed in that case. If the queue no longer exists, the Enqueue Exit as a priority message will return error 1. It is safe to ignore, because the module is already exiting."
            # "Another Module called the \"Stop Module\" API Method  or the Message Handling Loop below."
            n164 = event-data() -> ("Origin"=w71:string, "Exit via Stop Module Req?"=w67:bool, "Wait for Module to stop?"=w66:bool)  [unwired: 1 in]
            n165 = local write "Status"(w71) -> ()
            n166 = Bundle By Name(cluster=T5 {"Origin"="", "Exit via Stop Module Req?"=FALSE, "Wait for Module to stop?"=FALSE} ("Stop Argument"), "Exit via Stop Module Req?"=w67, "Wait for Module to stop?"=w66) -> (w65:T5)
            n167 = call-poly <vilib>:"Delacor_lib_QMH_Enqueue Message (poly).vi"("Priority Message? (F)"=TRUE, "Message Data"=w65, "Message"="Exit", "Message Queue in"=w72) -> ("error out"=w76:errorcluster)  [unwired: 6 in, 1 out]
            n168 = call <vilib>:"Clear Errors.vi"("error in (no error)"=w76, "specific error code to clear (0: all)"=1) -> ("error out"=w75:errorcluster)  [unwired: 4 in, 1 out]
          }
          event User Event {
            n169 = event-data() -> ()  [unwired: 1 in, 1 out]
            n170 = call-poly <vilib>:"Delacor_lib_QMH_Enqueue Message (poly).vi"("Message Data"="Conectando con la DAQ..." ("Message"), "Message"="Update status", "Message Queue in"=w80) -> ("error out"=w81:errorcluster, "Message Queue out"=w79:refnum<class "Delacor_lib_QMH_Message Queue.lvclass">)  [unwired: 7 in]
            n171 = call-poly <vilib>:"Delacor_lib_QMH_Enqueue Message (poly).vi"("error in"=w81, "Message"="Load config", "Message Queue in"=w79) -> ("error out"=w83:errorcluster)  [unwired: 7 in, 1 out]
          }
          event User Event {
            n172 = event-data() -> ()  [unwired: 1 in, 2 out]
            n173 = call-poly <vilib>:"Delacor_lib_QMH_Enqueue Message (poly).vi"("Message"="Configure DAQ", "Message Queue in"=w86) -> ("error out"=w87:errorcluster)  [unwired: 8 in, 1 out]
            "DAQ" <- TRUE ("DAQ")
          }
          event User Event {
            n174 = event-data() -> ("Data"=w89:dbl[])  [unwired: 1 in]
            n175 = Index Array(array=w89) -> (element=w88:dbl)  [unwired: 1 in]
            n176 = call-poly <vilib>:"Delacor_lib_QMH_Enqueue Message (poly).vi"("Message Data"=w88, "Message"="Update graph", "Message Queue in"=w91) -> ("error out"=w92:errorcluster)  [unwired: 7 in, 1 out]
          }
          event Panel Close? {
            w96 = TRUE  # Discard the event, the MHL is responsible for closing and stopping this VI.
            # "Hide the panel or send the 'Exit' message if the user clicks the 'X' on the module main VI panel."
            n177 = event-data() -> ()  [unwired: 1 in, 1 out]
            n178 = property on="Property Node" class="Module Admin"(reference=w94) -> ("Accessors:External Launch"=w93:bool)  [unwired: 1 in, 2 out]
            n179 = case shown="True" w93 {
              tunnel: w95 -> [_ w103]
              tunnel: [_ w104] -> w97
              frame True {
                # "If externally launched, clicking the 'X' hides the panel, but doesn't close it."
                n180 = control-ref of="This VI"() -> (w100:refnum<vi>)
                n181 = call "Hide VI Panel.vi"("VI"=w100) -> ("error out"=w98:errorcluster)  [unwired: 10 in]
                n182 = call "Status Updated.vi"("error in"=w98, "Status"="Panel hidden." ("format string")) -> ()  [unwired: 9 in, 1 out]
              }
              frame False {
                # "If run as a stand-alone VI, clicking the panel 'X' stops the VI."
                n183 = call-poly <vilib>:"Delacor_lib_QMH_Enqueue Message (poly).vi"("Priority Message? (F)"=TRUE, "Message"="Exit", "Message Queue in"=w103) -> ("error out"=w104:errorcluster)  [unwired: 7 in, 1 out]
              }
            }
            n184 = event-data ("Event Filter Node")("Discard?"=w96) -> ()  [unwired: 1 in, 1 out]
          }
          event "Exit Button": Value Change {
            n185 = event-data() -> ()  [unwired: 1 in, 1 out]
            n186 = call-poly <vilib>:"Delacor_lib_QMH_Enqueue Message (poly).vi"("Message Data"="Cerrando programa..." ("Message"), "Message"="Update status", "Message Queue in"=w110) -> ("error out"=w108:errorcluster, "Message Queue out"=w109:refnum<class "Delacor_lib_QMH_Message Queue.lvclass">)  [unwired: 7 in]
            n187 = call-poly <vilib>:"Delacor_lib_QMH_Enqueue Message (poly).vi"("error in"=w108, "Message Array"=string[] ["Close file reference", "Exit"] ("Message"), "Message Queue in"=w109) -> ("error out"=w111:errorcluster)  [unwired: 7 in, 1 out]
          }
          event "Settings Button": Value Change {
            n188 = event-data() -> ()  [unwired: 1 in, 1 out]
            n189 = call-poly <vilib>:"Delacor_lib_QMH_Enqueue Message (poly).vi"("Message"="Call config dialog", "Message Queue in"=w113) -> ("error out"=w114:errorcluster)  [unwired: 8 in, 1 out]
          }
          event "Acquire": Value Change {
            n190 = event-data() -> ()  [unwired: 1 in, 1 out]
            n191 = call-poly <vilib>:"Delacor_lib_QMH_Enqueue Message (poly).vi"("Message"="Start acquiring", "Message Queue in"=w116) -> ("error out"=w117:errorcluster)  [unwired: 8 in, 1 out]
          }
          event "Stop Button": Value Change {
            n192 = event-data() -> ()  [unwired: 1 in, 1 out]
            n193 = call-poly <vilib>:"Delacor_lib_QMH_Enqueue Message (poly).vi"("Message"="Stop acquisition", "Message Queue in"=w119) -> ("error out"=w120:errorcluster)  [unwired: 8 in, 1 out]
          }
          event "Log": Value Change {
            n194 = event-data() -> ("NewVal"=w124:bool)  [unwired: 1 in]
            n195 = case shown="False" w124 {
              tunnel: ["Close file reference" "Open file reference"] -> w121
              frame False {
              }
              frame True {
              }
            }
            n196 = call-poly <vilib>:"Delacor_lib_QMH_Enqueue Message (poly).vi"("Message"=w121, "Message Queue in"=w122) -> ("error out"=w123:errorcluster)  [unwired: 8 in, 1 out]
          }
        }
        n197 = call-dynamic "Delacor_lib_QMH_Error Handler - Event Handling Loop.vi"("error in"=w40, "Message Queue in"=w34) -> ("dup error in"=w39:errorcluster)  [unwired: 8 in, 1 out]
      }
    }
    frame Error {
      # "Synchronize Caller Events.vi will inform Start Module.vi that the module has launched and will let the code calling Start Module.vi register for broadcasts and would permit the caller receive the broadcast that an error occurred at launch time."
      n198 = call-dynamic "Delacor_lib_QMH_Release Message Queue.vi"("error in"=w466, "Message Queue"=w459) -> ("error out"=w465:errorcluster)  [unwired: 9 in]
      n199 = call "Synchronize Caller Events.vi"("Singleton Module Admin in"=w460) -> ("error out"=w467:errorcluster)  [unwired: 9 in, 1 out]
      n200 = call "Module Name--constant.vi"() -> ("Module Name"=w463:string)  [unwired: 11 in]
      n201 = call "Stop Module.vi"("Module ID"=w458) -> ()  [unwired: 10 in, 1 out]
      n202 = Format Into String(format string="An error occurred during initialization. %s is no longer running.", w463) -> (resulting string=w461:string)  [unwired: 2 in, 1 out]
      n203 = Merge Errors(w465, w467) -> (w468:errorcluster)
      n204 = call "Error Reported.vi"("Additional Information"=w461, "Error"=w468) -> ()  [unwired: 9 in, 1 out]
    }
  }
  n205 = Merge Errors(w20, w23) -> (w19:errorcluster)
  n206 = call "Close Module.vi"("error in"=w19, "Module Admin in"=w14) -> ("error out"=w21:errorcluster, "External Launch"=w7:bool, "Module Admin out"=w8:refnum<class "Delacor_lib_QMH_Module Admin.lvclass">)  [unwired: 7 in]
  n207 = Unregister For Events(event registration refnum=w13, error in=w21) -> (error out=w18:errorcluster)
  "error out" <- w18
  n208 = case "External Launch?" shown="True" w7 {
    tunnel: w18 -> [_ w469]
    frame False {
    }
    frame True {
      n209 = case shown="No Error" w469 {
        frame No Error {
          n210 = invoke on="Invoke Node" class="VI" method="FP.Close"() -> ()  [unwired: 3 in, 3 out]
        }
        frame Error {
          n211 = disable-structure shown="Default" {
            frame condition #0 (active) {
              n212 = invoke class="VI" method="FP.Open"("Activate"=TRUE ("Activate?")) -> ()  [unwired: 4 in, 5 out]
            }
            frame condition #1 {
              # "Don't show panel on error if running inside a built EXE."
            }
          }
        }
      }
    }
  }
  n213 = local write "Module Admin"(w8) -> ()
